vi "From DateTime Array.vi"(1 "DateTime Array":timestamp[](array[timestamp])) -> (0 "Formatted DateTime Array":dbl[](array[numeric]))   [LabVIEW 2013, in "OPC UA Server runtime.lvclass"]
doc: "Convert DateTime array to a data type which can be used by DCAF"
uses:
  OPC UA Server runtime.lvclass
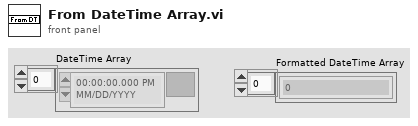
[diagram p1: front panel]
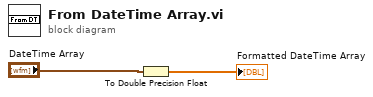
[diagram p0: block diagram]
diagram:
  n1 = To Double Precision Float(number="DateTime Array") -> (double precision float=→"Formatted DateTime Array":dbl[])
